vi "Normalize.vi"(4 "Focus Curve In":cluster{"Z (um)":dbl[], "Score":sgl[]}) -> (0 "min":sgl, 1 "Focus Curve Out":cluster{"Z (um)":dbl[], "Score":sgl[]}, 2 "max":sgl)   [LabVIEW 2014]
panel:
  # "LICENSED MATERIALS – PROPERTY OF IBM\nCopyright IBM Corp. 2016,\nALL RIGHTS RESERVED"
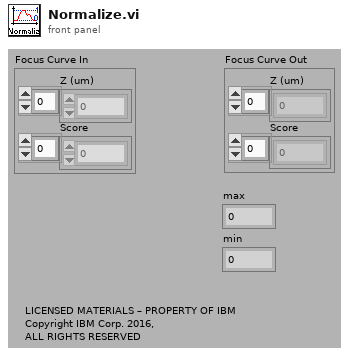
[diagram p1: front panel]
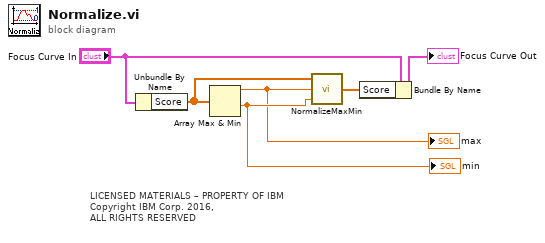
[diagram p0: block diagram]
diagram:
  # "LICENSED MATERIALS – PROPERTY OF IBM\nCopyright IBM Corp. 2016,\nALL RIGHTS RESERVED"
  n1 = Unbundle By Name("Focus Curve In") -> ("Score"=w6:sgl[])
  n2 = Array Max & Min(array=w6) -> (max value=w1:sgl, min value=w2:sgl)  [unwired: 2 out]
  "max" <- w1
  "min" <- w2
  n3 = call "NormalizeMaxMin.vi"("Min"=w2, "Max"=w1, "Score"=w6) -> ("Array"=w3:sgl[])
  n4 = Bundle By Name(cluster="Focus Curve In", "Score"=w3) -> (→"Focus Curve Out":cluster{"Z (um)":dbl[], "Score":sgl[]})
